vi "ASI Get Control Caps.vi"(9 "pControlCaps":T1 {"IsAutoSupported" items=["ASI_FALSE", "ASI_TRUE"]; "IsWritable" items=["ASI_FALSE", "ASI_TRUE"]; "ControlType" items=["ASI_GAIN", "ASI_EXPOSURE", "ASI_GAMMA", "ASI_WB_R", "ASI_WB_B", "ASI_BRIGHTNESS", "ASI_BANDWIDTHOVERLOAD", "ASI_OVERCLOCK", "ASI_TEMPERATURE", "ASI_FLIP", "ASI_AUTO_MAX_GAIN", "ASI_AUTO_MAX_EXP", "ASI_AUTO_MAX_BRIGHTNESS", "ASI_HARDWARE_BIN", "ASI_HIGH_SPEED_MODE", "ASI_COOLER_POWER_PERC", "ASI_TARGET_TEMP", "ASI_COOLER_ON", "ASI_MONO_BIN", "ASI_FAN_ON", "ASI_PATTERN_ADJUST", "ASI_ANTI_DEW_HEATER", "ASI_AUTO_MAX_EXP_MS"]}, 10 "iControlIndex":i32, 11 "iCameraID":i32) -> (0 "name":string, 1 "pControlCaps out":T1 {"IsAutoSupported" items=["ASI_FALSE", "ASI_TRUE"]; "IsWritable" items=["ASI_FALSE", "ASI_TRUE"]; "ControlType" items=["ASI_GAIN", "ASI_EXPOSURE", "ASI_GAMMA", "ASI_WB_R", "ASI_WB_B", "ASI_BRIGHTNESS", "ASI_BANDWIDTHOVERLOAD", "ASI_OVERCLOCK", "ASI_TEMPERATURE", "ASI_FLIP", "ASI_AUTO_MAX_GAIN", "ASI_AUTO_MAX_EXP", "ASI_AUTO_MAX_BRIGHTNESS", "ASI_HARDWARE_BIN", "ASI_HIGH_SPEED_MODE", "ASI_COOLER_POWER_PERC", "ASI_TARGET_TEMP", "ASI_COOLER_ON", "ASI_MONO_BIN", "ASI_FAN_ON", "ASI_PATTERN_ADJUST", "ASI_ANTI_DEW_HEATER", "ASI_AUTO_MAX_EXP_MS"]}, 3 "function return":i32)   [LabVIEW 2023, in "ASICamera2_no_err.lvlib"]
doc: "ASICAMERA_API ASI_ERROR_CODE ASIGetControlCaps(int iCameraID, int iControlIndex, ASI_CONTROL_CAPS * pControlCaps);"
uses:
  ASICamera2_no_err.lvlib
  LabviewDAQ-master/ConcreteClasses/ConcreteInstrumentClasses/CameraClasses/ZWO_ASI_LV/Labview_ASI_demo_64bit_221128/user.lib/ASICamera2_no_err/ASICamera2.dll
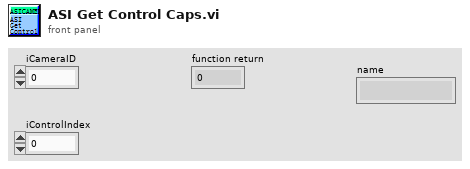
[diagram p1: front panel]
types:
  T1 = cluster{"Name[0]":i8, "Name[1]":i8, "Name[2]":i8, "Name[3]":i8, "Name[4]":i8, "Name[5]":i8, "Name[6]":i8, "Name[7]":i8, "Name[8]":i8, "Name[9]":i8, "Name[10]":i8, "Name[11]":i8, "Name[12]":i8, "Name[13]":i8, "Name[14]":i8, "Name[15]":i8, "Name[16]":i8, "Name[17]":i8, "Name[18]":i8, "Name[19]":i8, "Name[20]":i8, "Name[21]":i8, "Name[22]":i8, "Name[23]":i8, "Name[24]":i8, "Name[25]":i8, "Name[26]":i8, "Name[27]":i8, "Name[28]":i8, "Name[29]":i8, "Name[30]":i8, "Name[31]":i8, "Name[32]":i8, "Name[33]":i8, "Name[34]":i8, "Name[35]":i8, "Name[36]":i8, "Name[37]":i8, "Name[38]":i8, "Name[39]":i8, "Name[40]":i8, "Name[41]":i8, "Name[42]":i8, "Name[43]":i8, "Name[44]":i8, "Name[45]":i8, "Name[46]":i8, "Name[47]":i8, "Name[48]":i8, "Name[49]":i8, "Name[50]":i8, "Name[51]":i8, "Name[52]":i8, "Name[53]":i8, "Name[54]":i8, "Name[55]":i8, "Name[56]":i8, "Name[57]":i8, "Name[58]":i8, "Name[59]":i8, "Name[60]":i8, "Name[61]":i8, "Name[62]":i8, "Name[63]":i8, "Description[0]":i8, "Description[1]":i8, "Description[2]":i8, "Description[3]":i8, "Description[4]":i8, "Description[5]":i8, "Description[6]":i8, "Description[7]":i8, "Description[8]":i8, "Description[9]":i8, "Description[10]":i8, "Description[11]":i8, "Description[12]":i8, "Description[13]":i8, "Description[14]":i8, "Description[15]":i8, "Description[16]":i8, "Description[17]":i8, "Description[18]":i8, "Description[19]":i8, "Description[20]":i8, "Description[21]":i8, "Description[22]":i8, "Description[23]":i8, "Description[24]":i8, "Description[25]":i8, "Description[26]":i8, "Description[27]":i8, "Description[28]":i8, "Description[29]":i8, "Description[30]":i8, "Description[31]":i8, "Description[32]":i8, "Description[33]":i8, "Description[34]":i8, "Description[35]":i8, "Description[36]":i8, "Description[37]":i8, "Description[38]":i8, "Description[39]":i8, "Description[40]":i8, "Description[41]":i8, "Description[42]":i8, "Description[43]":i8, "Description[44]":i8, "Description[45]":i8, "Description[46]":i8, "Description[47]":i8, "Description[48]":i8, "Description[49]":i8, "Description[50]":i8, "Description[51]":i8, "Description[52]":i8, "Description[53]":i8, "Description[54]":i8, "Description[55]":i8, "Description[56]":i8, "Description[57]":i8, "Description[58]":i8, "Description[59]":i8, "Description[60]":i8, "Description[61]":i8, "Description[62]":i8, "Description[63]":i8, "Description[64]":i8, "Description[65]":i8, "Description[66]":i8, "Description[67]":i8, "Description[68]":i8, "Description[69]":i8, "Description[70]":i8, "Description[71]":i8, "Description[72]":i8, "Description[73]":i8, "Description[74]":i8, "Description[75]":i8, "Description[76]":i8, "Description[77]":i8, "Description[78]":i8, "Description[79]":i8, "Description[80]":i8, "Description[81]":i8, "Description[82]":i8, "Description[83]":i8, "Description[84]":i8, "Description[85]":i8, "Description[86]":i8, "Description[87]":i8, "Description[88]":i8, "Description[89]":i8, "Description[90]":i8, "Description[91]":i8, "Description[92]":i8, "Description[93]":i8, "Description[94]":i8, "Description[95]":i8, "Description[96]":i8, "Description[97]":i8, "Description[98]":i8, "Description[99]":i8, "Description[100]":i8, "Description[101]":i8, "Description[102]":i8, "Description[103]":i8, "Description[104]":i8, "Description[105]":i8, "Description[106]":i8, "Description[107]":i8, "Description[108]":i8, "Description[109]":i8, "Description[110]":i8, "Description[111]":i8, "Description[112]":i8, "Description[113]":i8, "Description[114]":i8, "Description[115]":i8, "Description[116]":i8, "Description[117]":i8, "Description[118]":i8, "Description[119]":i8, "Description[120]":i8, "Description[121]":i8, "Description[122]":i8, "Description[123]":i8, "Description[124]":i8, "Description[125]":i8, "Description[126]":i8, "Description[127]":i8, "MaxValue":i32, "MinValue":i32, "DefaultValue":i32, "IsAutoSupported":u32, "IsWritable":u32, "ControlType":u32, "Unused[0]":i8, "Unused[1]":i8, "Unused[2]":i8, "Unused[3]":i8, "Unused[4]":i8, "Unused[5]":i8, "Unused[6]":i8, "Unused[7]":i8, "Unused[8]":i8, "Unused[9]":i8, "Unused[10]":i8, "Unused[11]":i8, "Unused[12]":i8, "Unused[13]":i8, "Unused[14]":i8, "Unused[15]":i8, "Unused[16]":i8, "Unused[17]":i8, "Unused[18]":i8, "Unused[19]":i8, "Unused[20]":i8, "Unused[21]":i8, "Unused[22]":i8, "Unused[23]":i8, "Unused[24]":i8, "Unused[25]":i8, "Unused[26]":i8, "Unused[27]":i8, "Unused[28]":i8, "Unused[29]":i8, "Unused[30]":i8, "Unused[31]":i8}
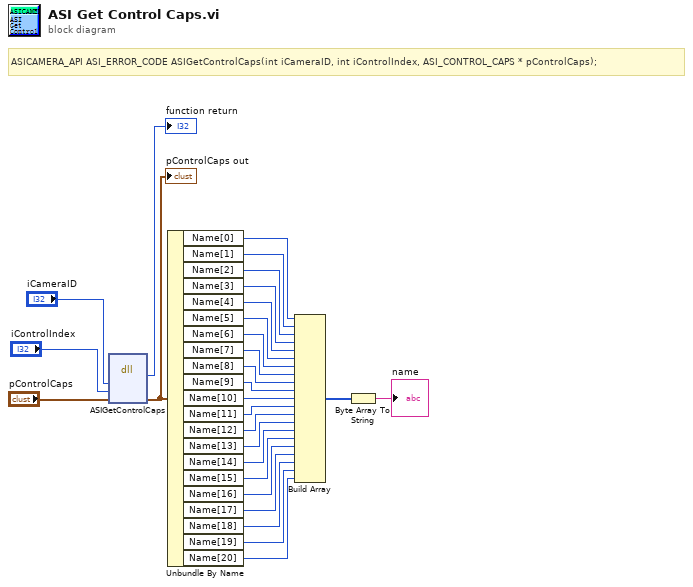
[diagram p0: block diagram]
diagram:
  # "ASICAMERA_API ASI_ERROR_CODE ASIGetControlCaps(int iCameraID, int iControlIndex, ASI_CONTROL_CAPS * pControlCaps);"
  n1 = dll-call lib="W:/Quant_Opt_Group/Group/Alex/LabviewDAQ-master/ConcreteClasses/ConcreteInstrumentClasses/CameraClasses/ZWO_ASI_LV/Labview_ASI_demo_64bit_221128/user.lib/ASICamera2_no_err/ASICamera2.*" fn="ASIGetControlCaps"("iCameraID"="iCameraID", "iControlIndex"="iControlIndex", "pControlCaps"="pControlCaps") -> (→"function return":i32, "pControlCaps"=w24:T1)  [unwired: 5 in, 2 out]
  "pControlCaps out" <- w24
  n2 = Unbundle By Name(w24) -> ("Name[0]"=w23:i8, "Name[1]"=w22:i8, "Name[2]"=w21:i8, "Name[3]"=w20:i8, "Name[4]"=w19:i8, "Name[5]"=w18:i8, "Name[6]"=w17:i8, "Name[7]"=w16:i8, "Name[8]"=w15:i8, "Name[9]"=w14:i8, "Name[10]"=w13:i8, "Name[11]"=w12:i8, "Name[12]"=w11:i8, "Name[13]"=w10:i8, "Name[14]"=w9:i8, "Name[15]"=w8:i8, "Name[16]"=w7:i8, "Name[17]"=w6:i8, "Name[18]"=w5:i8, "Name[19]"=w4:i8, "Name[20]"=w3:i8)
  n3 = Build Array(w23, w22, w21, w20, w19, w18, w17, w16, w15, w14, w13, w12, w11, w10, w9, w8, w7, w6, w5, w4, w3) -> (w2:i8[])
  n4 = Byte Array To String(unsigned byte array=w2) -> (string=→"name":string)
